vi "AcquireWaveformNotXYPair.vi"(8 "error in (no error)":errorcluster, 9 "Measurement (Ch1)":i32, 10 "Instrument Handle In":i32, 11 "Data in":T1={"DAQ Config Data"={"Vertical"={"Coupling"=0, "Offset (V)"=0.0, "Range (V)"=0.0, "Impedance"=0.0}, "Horizontal"={"Offset Time"=0.0, "Sample Time (S)"=0.0, "Sample Points"=0}, "Trigger\n"={"Lower Level (V)"=0.0, "Trigger Slope"=0, "Trigger Source"=0}, "Acquisition"={"Trigger Mode"=0, "Initiate Continuously"=0, "Acquire Type"=0, "Acquire Count"=1}, "Channel"=0, "Instrument Handle"=0, "Error"={"status"=FALSE, "code"=0, "source"=""}, "State"=0}, "Acquisition"={"Current"={"Acquiring Now?"=FALSE, "Waveforms Acquired"=0.0, "Start of Acquisition"=timestamp(0 s since 1904-01-01), "Acquisition Name"=""}, "Stop Condition"={"Quota"=0.0, "Duration (S)"=0, "Stop Condition"=FALSE}, "Config Needed"=FALSE}, "Measurement"={"Waveform"={"t0"=timestamp(0 s since 1904-01-01), "dt"=1.0, "Y"=[]}, "Peak Heights"=[], "Acquisition Time"=timestamp(0 s since 1904-01-01), "File Path"=path "C:/Users/lab-341/Desktop/Reed/Oscilloscope VI/pulses.tdms", "TDMS File Handle"=refnum}, "UI References"={"Acquire"=refnum, "Configure DAQ"=refnum, "Measurement (Ch1)"=refnum, "Update Needed?"=FALSE, "New Run"=refnum, "Signal"=refnum}, "Run Info"={"Active Run?"=FALSE, "Run Notes"="Enter in notes explaining the purpose of the run and any unusual steps taken in the process. This should make it clear why the data was taken. e.g. \"Measuring LXe scintillation light with Teflon\" or \"Measuring dark pulses to determine SPE gain.\" Concise is good but precise is better.", "User Name"="", "Campaign ID#"="", "Run Name"="", "Start Time"=timestamp(0 s since 1904-01-01), "End Time"=timestamp(0 s since 1904-01-01)}, "System Status"={"Bias Voltage"=0.0, "SiPM Temperature"=[], "Slow Control User"="", "LXe"=0.0}, "Acquisition Info"={"Trigger Mode"=FALSE, "Acquisition Mode"=FALSE, "Bias Voltage (V)"=0.0, "Preamplifier"=0, "Shaping Amplifier"=0, "Acquisition Notes"="", "1"=FALSE, "2"=FALSE}} {"Acquisition Info"."Shaping Amplifier" items=["CR-200-100ns", "CR-200-1us"]; "Acquisition Info"."Preamplifier" items=["CR-Z-113-1k", "CR-Z-113-5k", "CR-Z-SiPM"]; "DAQ Config Data"."State" items=["Enable"=1, "Disable"=0]; "DAQ Config Data"."Channel" items=["Input Channel 1", "Input Channel 2", "Input Channel 3", "Input Channel 4"]; "DAQ Config Data"."Acquisition"."Acquire Type" items=["Normal"=0, "Average"=1, "Envelope"=2, "Peak Detect"=3, "High Resolution"=4, "Fast"=5, "Equivalent Time"=16]; "DAQ Config Data"."Acquisition"."Initiate Continuously" items=["Continuously"=1, "Single Capture"=0]; "DAQ Config Data"."Acquisition"."Trigger Mode" items=["Auto", "Normal"]; "DAQ Config Data"."Trigger"."Trigger Source" items=["TTL0", "TTL1", "TTL2", "TTL3", "TTL4", "TTL5", "TTL6", "TTL7", "ECL0", "ECL1", "Input Channel 1", "Input Channel 2", "Input Channel 3", "Input Channel 4", "External Trigger Source", "STAR", "Manual Trigger", "Pattern"]; "DAQ Config Data"."Trigger"."Trigger Slope" items=["Rising Edge", "Falling Edge"]; "DAQ Config Data"."Horizontal"."Sample Time (S)" items=["0.5"=0.5, "0.4"=0.4, "0.25"=0.25, "0.2"=0.2, "0.1"=0.1, "0.05"=0.05, "0.04"=0.04, "0.025"=0.025, "0.02"=0.02, "0.01"=0.01, "0.005"=0.005, "0.004"=0.004, "0.0025"=0.0025, "0.002"=0.002, "0.001"=0.001, "5E-4"=0.0005, "4E-4"=0.0004, "2.5E-4"=0.00025, "2E-4"=0.0002, "1E-4"=0.0001, "5E-5"=5e-05, "4E-5"=4e-05, "2E-5"=2e-05, "5E-6"=5e-06, "1E-6"=1e-06, "5E-7"=5e-07, "1E-7"=1e-07, "5E-8"=5e-08, "1E-8"=1e-08]; "DAQ Config Data"."Vertical"."Impedance" items=["50 Ohm"=50.0, "1 MOhm"=1000000.0]; "DAQ Config Data"."Vertical"."Range (V)" items=["10"=10.0, "5"=5.0, "2"=2.0, "1"=1.0, "0.4"=0.4, "0.2"=0.2, "0.08"=0.08, "0.04"=0.04, "0.02"=0.02, "0.01"=0.01]; "DAQ Config Data"."Vertical"."Coupling" items=["AC", "DC"]}) -> (0 "error out":errorcluster, 2 "Instrument Handle Out":i32, 3 "Data out":T1={"DAQ Config Data"={"Vertical"={"Coupling"=0, "Offset (V)"=0.0, "Range (V)"=0.0, "Impedance"=0.0}, "Horizontal"={"Offset Time"=0.0, "Sample Time (S)"=0.0, "Sample Points"=0}, "Trigger\n"={"Lower Level (V)"=0.0, "Trigger Slope"=0, "Trigger Source"=0}, "Acquisition"={"Trigger Mode"=0, "Initiate Continuously"=0, "Acquire Type"=0, "Acquire Count"=1}, "Channel"=0, "Instrument Handle"=0, "Error"={"status"=FALSE, "code"=0, "source"=""}, "State"=0}, "Acquisition"={"Current"={"Acquiring Now?"=FALSE, "Waveforms Acquired"=0.0, "Start of Acquisition"=timestamp(0 s since 1904-01-01), "Acquisition Name"=""}, "Stop Condition"={"Quota"=0.0, "Duration (S)"=0, "Stop Condition"=FALSE}, "Config Needed"=FALSE}, "Measurement"={"Waveform"={"t0"=timestamp(0 s since 1904-01-01), "dt"=1.0, "Y"=[]}, "Peak Heights"=[], "Acquisition Time"=timestamp(0 s since 1904-01-01), "File Path"=path "C:/Users/lab-341/Desktop/Reed/Oscilloscope VI/pulses.tdms", "TDMS File Handle"=refnum}, "UI References"={"Acquire"=refnum, "Configure DAQ"=refnum, "Measurement (Ch1)"=refnum, "Update Needed?"=FALSE, "New Run"=refnum, "Signal"=refnum}, "Run Info"={"Active Run?"=FALSE, "Run Notes"="Enter in notes explaining the purpose of the run and any unusual steps taken in the process. This should make it clear why the data was taken. e.g. \"Measuring LXe scintillation light with Teflon\" or \"Measuring dark pulses to determine SPE gain.\" Concise is good but precise is better.", "User Name"="", "Campaign ID#"="", "Run Name"="", "Start Time"=timestamp(0 s since 1904-01-01), "End Time"=timestamp(0 s since 1904-01-01)}, "System Status"={"Bias Voltage"=0.0, "SiPM Temperature"=[], "Slow Control User"="", "LXe"=0.0}, "Acquisition Info"={"Trigger Mode"=FALSE, "Acquisition Mode"=FALSE, "Bias Voltage (V)"=0.0, "Preamplifier"=0, "Shaping Amplifier"=0, "Acquisition Notes"="", "1"=FALSE, "2"=FALSE}} {"Acquisition Info"."Shaping Amplifier" items=["CR-200-100ns", "CR-200-1us"]; "Acquisition Info"."Preamplifier" items=["CR-Z-113-1k", "CR-Z-113-5k", "CR-Z-SiPM"]; "DAQ Config Data"."State" items=["Enable"=1, "Disable"=0]; "DAQ Config Data"."Channel" items=["Input Channel 1", "Input Channel 2", "Input Channel 3", "Input Channel 4"]; "DAQ Config Data"."Acquisition"."Acquire Type" items=["Normal"=0, "Average"=1, "Envelope"=2, "Peak Detect"=3, "High Resolution"=4, "Fast"=5, "Equivalent Time"=16]; "DAQ Config Data"."Acquisition"."Initiate Continuously" items=["Continuously"=1, "Single Capture"=0]; "DAQ Config Data"."Acquisition"."Trigger Mode" items=["Auto", "Normal"]; "DAQ Config Data"."Trigger"."Trigger Source" items=["TTL0", "TTL1", "TTL2", "TTL3", "TTL4", "TTL5", "TTL6", "TTL7", "ECL0", "ECL1", "Input Channel 1", "Input Channel 2", "Input Channel 3", "Input Channel 4", "External Trigger Source", "STAR", "Manual Trigger", "Pattern"]; "DAQ Config Data"."Trigger"."Trigger Slope" items=["Rising Edge", "Falling Edge"]; "DAQ Config Data"."Horizontal"."Sample Time (S)" items=["0.5"=0.5, "0.4"=0.4, "0.25"=0.25, "0.2"=0.2, "0.1"=0.1, "0.05"=0.05, "0.04"=0.04, "0.025"=0.025, "0.02"=0.02, "0.01"=0.01, "0.005"=0.005, "0.004"=0.004, "0.0025"=0.0025, "0.002"=0.002, "0.001"=0.001, "5E-4"=0.0005, "4E-4"=0.0004, "2.5E-4"=0.00025, "2E-4"=0.0002, "1E-4"=0.0001, "5E-5"=5e-05, "4E-5"=4e-05, "2E-5"=2e-05, "5E-6"=5e-06, "1E-6"=1e-06, "5E-7"=5e-07, "1E-7"=1e-07, "5E-8"=5e-08, "1E-8"=1e-08]; "DAQ Config Data"."Vertical"."Impedance" items=["50 Ohm"=50.0, "1 MOhm"=1000000.0]; "DAQ Config Data"."Vertical"."Range (V)" items=["10"=10.0, "5"=5.0, "2"=2.0, "1"=1.0, "0.4"=0.4, "0.2"=0.2, "0.08"=0.08, "0.04"=0.04, "0.02"=0.02, "0.01"=0.01]; "DAQ Config Data"."Vertical"."Coupling" items=["AC", "DC"]})   [LabVIEW 2023]
uses:
  TypeDefs/DataTypes/Data.ctl
  TypeDefs/DataTypes/DAQConfig.ctl
  TypeDefs/DataTypes/Acquisition.ctl
  TypeDefs/DataTypes/Current.ctl
  TypeDefs/DataTypes/StopCondition.ctl
  TypeDefs/DataTypes/Measurement.ctl
  TypeDefs/DataTypes/UIReferences.ctl
  TypeDefs/DataTypes/RunInfo.ctl
  TypeDefs/DataTypes/SystemStatus.ctl
panel:
  # "Shaper Gain"
  # "Self"
  # "Fast"
  # "Solicited"
  # "Standard"
  # "Shaper Gain"
  # "Self"
  # "Fast"
  # "Solicited"
  # "Standard"
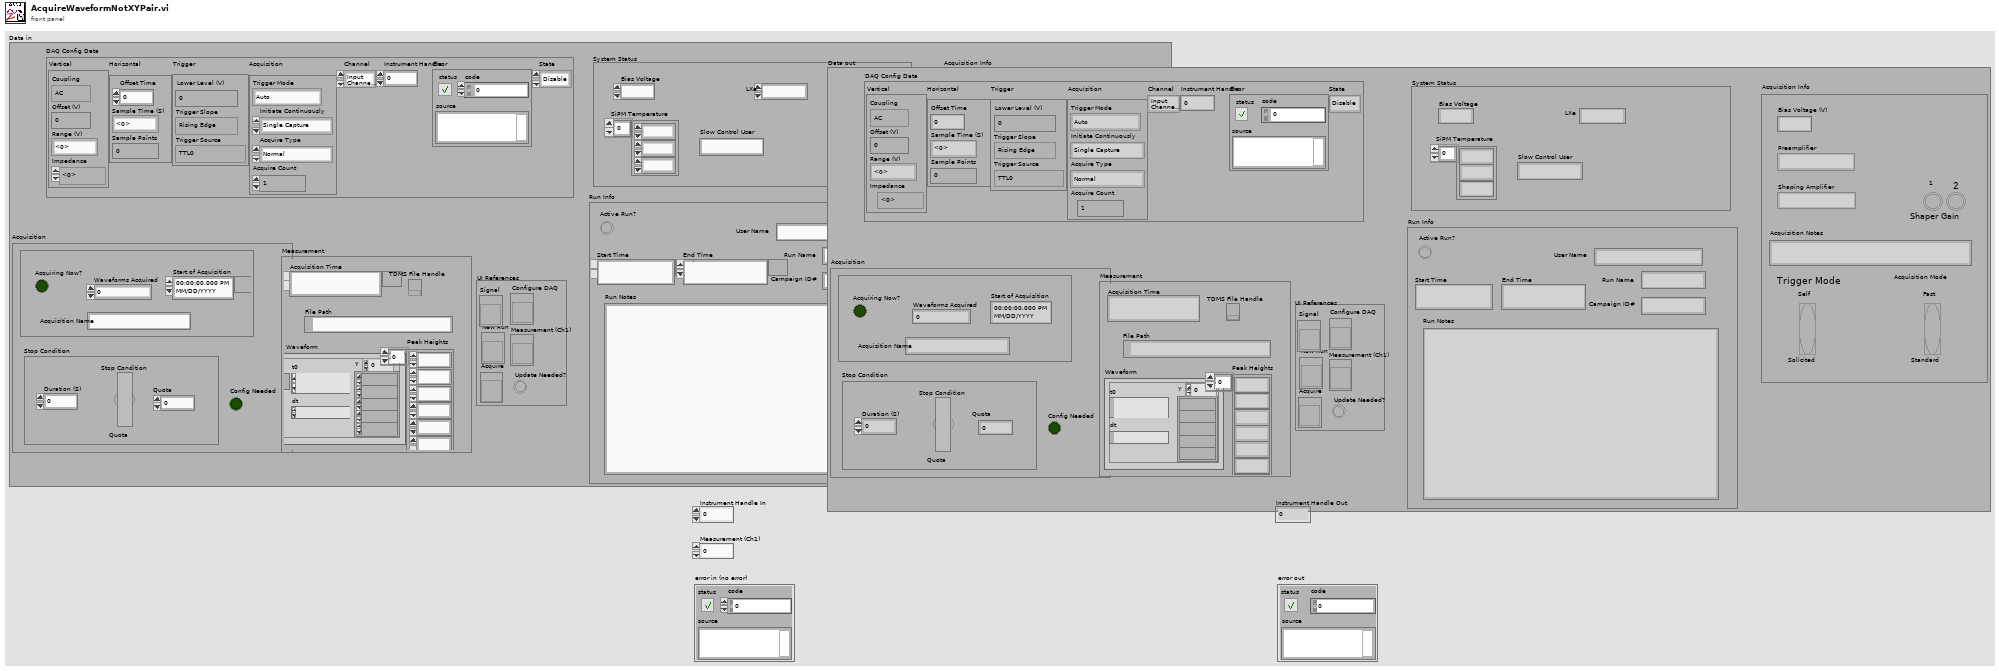
[diagram p1: front panel]
types:
  T1 = typedef "Data.ctl" = cluster{"DAQ Config Data":T2, "Acquisition":T3, "Measurement":T6, "UI References":T7, "Run Info":T8, "System Status":T9, "Acquisition Info":cluster{"Trigger Mode":bool, "Acquisition Mode":bool, "Bias Voltage (V)":dbl, "Preamplifier":u16, "Shaping Amplifier":u16, "Acquisition Notes":string, "1":bool, "2":bool}}
  T2 = typedef "DAQConfig.ctl" = cluster{"Vertical":cluster{"Coupling":i32, "Offset (V)":dbl, "Range (V)":dbl, "Impedance":dbl}, "Horizontal":cluster{"Offset Time":dbl, "Sample Time (S)":dbl, "Sample Points":u32}, "Trigger\n":cluster{"Lower Level (V)":dbl, "Trigger Slope":i32, "Trigger Source":i32}, "Acquisition":cluster{"Trigger Mode":i32, "Initiate Continuously":i32, "Acquire Type":i32, "Acquire Count":i32}, "Channel":i32, "Instrument Handle":i32, "Error":errorcluster, "State":i32}
  T3 = typedef "Acquisition.ctl" = cluster{"Current":T4, "Stop Condition":T5, "Config Needed":bool}
  T4 = typedef "Current.ctl" = cluster{"Acquiring Now?":bool, "Waveforms Acquired":dbl, "Start of Acquisition":timestamp, "Acquisition Name":string}
  T5 = typedef "StopCondition.ctl" = cluster{"Quota":dbl, "Duration (S)":u16, "Stop Condition":bool}
  T6 = typedef "Measurement.ctl" = cluster{"Waveform":waveform(dbl), "Peak Heights":dbl[], "Acquisition Time":timestamp, "File Path":path, "TDMS File Handle":refnum<k34>}
  T7 = typedef "UIReferences.ctl" = cluster{"Acquire":refnum<vi>, "Configure DAQ":refnum<vi>, "Measurement (Ch1)":refnum<vi>, "Update Needed?":bool, "New Run":refnum<vi>, "Signal":refnum<vi>}
  T8 = typedef "RunInfo.ctl" = cluster{"Active Run?":bool, "Run Notes":string, "User Name":string, "Campaign ID#":string, "Run Name":string, "Start Time":timestamp, "End Time":timestamp}
  T9 = typedef "SystemStatus.ctl" = cluster{"Bias Voltage":dbl, "SiPM Temperature":dbl[], "Slow Control User":string, "LXe":dbl}
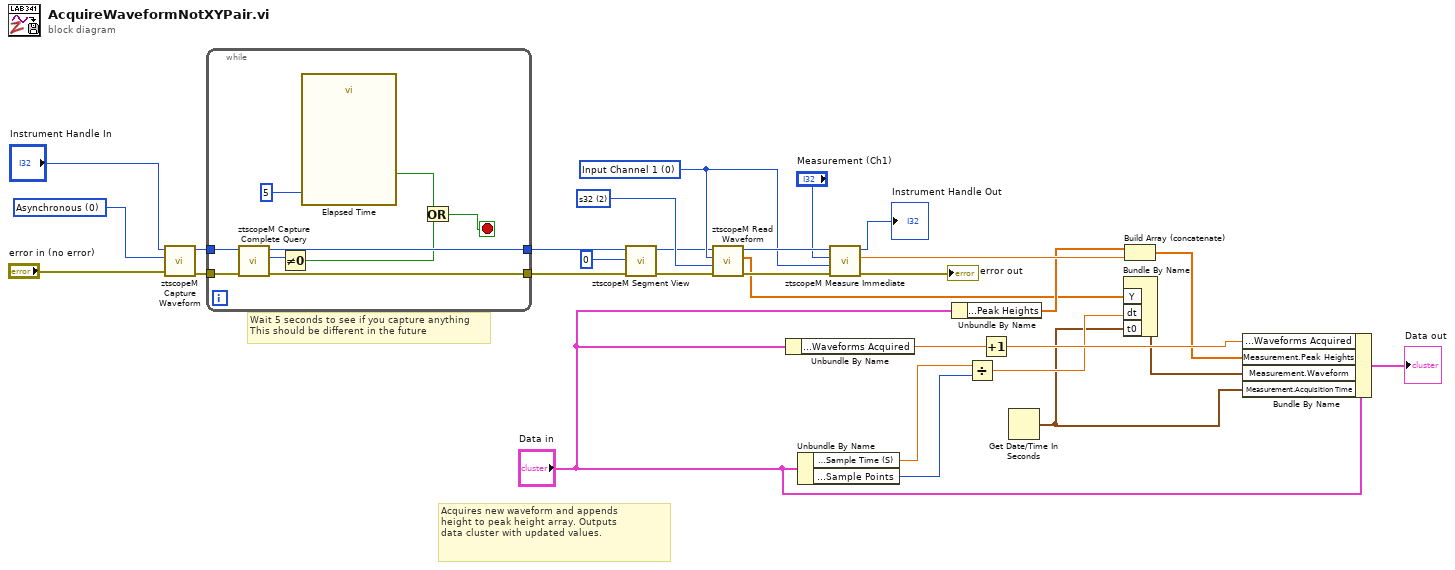
[diagram p0: block diagram]
diagram:
  w24 = 0 items=["Input Channel 1", "Input Channel 2", "Input Channel 3", "Input Channel 4", "Calc Channel 1", "Calc Channel 2", "Calc Channel 3", "Calc Channel 4", "Ref Channel 1", "Ref Channel 2", "Ref Channel 3", "Ref Channel 4"] ("Source")
  w22 = 2 items=["s8", "s16", "s32", "f32", "f64"] ("Transfer Type")
  w16 = 0 items=["Infinite"=-1, "Asynchronous"=0] ("Timeout")
  # "Wait 5 seconds to see if you capture anything\nThis should be different in the future"
  # "Acquires new waveform and appends\nheight to peak height array. Outputs\ndata cluster with updated values."
  n1 = call <instrlib>:"ztscopeM Capture Waveform.vi"("error in"="error in (no error)", "Timeout"=w16, "Instrument Handle In"="Instrument Handle In") -> ("error out"=w4:errorcluster, "Instrument Handle Out"=w3:i32)  [unwired: 7 in]
  n2 = while {
    tunnel: w3 -> [w39]
    tunnel: [w37] -> w2
    tunnel: w4 -> [w36]
    tunnel: [w35] -> w1
    stop <- w31 stop-if-true
    n3 = call <instrlib>:"ztscopeM Capture Complete Query.vi"("error in"=w36, "Instrument Handle In"=w39) -> ("error out"=w35:errorcluster, "State"=w38:i32, "Instrument Handle Out"=w37:i32)  [unwired: 7 in]
    n4 = Not Equal To 0?(x=w38) -> (x != 0?=w32:bool)
    n5 = call "Elapsed Time"("Time Target (s)"=5 ("Timeout")) -> ("Time has Elapsed"=w33:bool)  [unwired: 11 in, 7 out]
    n6 = Or(x=w33, y=w32) -> (x .or. y?=w31:bool)
  }
  n7 = call <instrlib>:"ztscopeM Segment View.vi"("error in"=w1, "Segment Number"=0, "Instrument Handle In"=w2) -> ("error out"=w20:errorcluster, "Instrument Handle Out"=w19:i32)  [unwired: 7 in]
  n8 = call <instrlib>:"ztscopeM Read Waveform.vi"("error in"=w20, "Transfer Type"=w22, "Source"=w24, "Instrument Handle In"=w19) -> ("error out"=w25:errorcluster, "Waveform"=w12:dbl[], "Instrument Handle Out"=w27:i32)  [unwired: 4 in, 1 out]
  n9 = Unbundle By Name("Data in") -> ("Acquisition.Current.Waveforms Acquired"=w15:dbl)
  n10 = Unbundle By Name("Data in") -> ("DAQ Config Data.Horizontal.Sample Time (S)"=w10:dbl, "DAQ Config Data.Horizontal.Sample Points"=w9:u32)
  n11 = call <instrlib>:"ztscopeM Measure Immediate.vi"("error in"=w25, "Source"=w24, "Measurement"="Measurement (Ch1)", "Instrument Handle In"=w27) -> ("error out"=→"error out":errorcluster, "Result"=w30:dbl, "Instrument Handle Out"=→"Instrument Handle Out":i32)  [unwired: 5 in]
  n12 = Unbundle By Name("Data in") -> ("Measurement.Peak Heights"=w29:dbl[])
  n13 = Divide(x=w10, y=w9) -> (x/y=w8:dbl)
  n14 = Increment(x=w15) -> (x+1=w14:dbl)
  n15 = Get Date/Time In Seconds() -> (seconds since 1Jan1904=w7:timestamp)
  n16 = Bundle By Name("Y"=w12, "dt"=w8, "t0"=w7) -> (w5:waveform(dbl))  [unwired: 1 in]
  n17 = Build Array (concatenate)(w29, w30) -> (w6:dbl[])
  n18 = Bundle By Name(cluster="Data in", "Acquisition.Current.Waveforms Acquired"=w14, "Measurement.Peak Heights"=w6, "Measurement.Waveform"=w5, "Measurement.Acquisition Time"=w7) -> (→"Data out":T1)
